vi "AprilTagFieldLayout_New2024.vi"() -> (3 "AprilTagFieldLayout":T1={"AprilTagMap"={}, "FieldLength"=0.0, "FieldWidth"=0.0, "OriginPosition "=enum."kBlueAllianceWallRightSide,", "OriginPose3d"={"Translation3d"={"X"=0.0, "Y"=0.0, "Z"=0.0}, "Rotation3d"={"Q_quaternion"={"R"=1.0, "V"=[0.0, 0.0, 0.0]}}}} {"OriginPose3d"."Translation3d"."Z" format="%14.3f"; "OriginPose3d"."Translation3d"."Y" format="%14.3f"; "OriginPose3d"."Translation3d"."X" format="%14.3f"})   [LabVIEW 2019, in "Trajectory_Library.lvlib"]
doc: "Define the FRC 2024 April Tag field layout.\n\nInputs:\n <none>\n\nOutputs:\n -- AprilTagFieldLayout -- AprilTagFieldLayout -- Data cluster containing field definition."
uses:
  Trajectory_Library.lvlib
  TypeDef/AprilTagFieldLayout.ctl
  TypeDef/AprilTag.ctl
  TypeDef/POSE3D.ctl
  TypeDef/TRANSLATION3D.ctl
  TypeDef/ROTATION3D.ctl
  TypeDef/QUATERNION.ctl
  Enum/AprilTagFieldLayoutOrignPosition_ENUM.ctl
  AprilTag_GetAll.vi
  Quaternion_Normalize.vi
  Quaternion_New_Default.vi
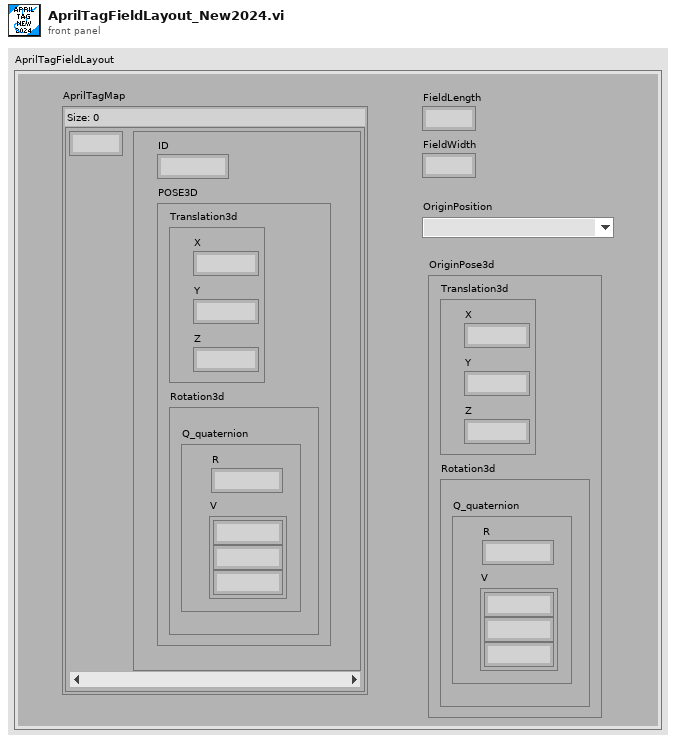
[diagram p1: front panel]
types:
  T1 = typedef "Trajectory_Library.lvlib/AprilTagFieldLayout.ctl" = cluster{"AprilTagMap":map{i32, T2}, "FieldLength":dbl, "FieldWidth":dbl, "OriginPosition ":T7, "OriginPose3d":T3}
  T2 = typedef "Trajectory_Library.lvlib/AprilTag.ctl" = cluster{"ID":i32, "POSE3D":T3}
  T3 = typedef "Trajectory_Library.lvlib/POSE3D.ctl" = cluster{"Translation3d":T4, "Rotation3d":T5}
  T4 = typedef "Trajectory_Library.lvlib/TRANSLATION3D.ctl" = cluster{"X":dbl, "Y":dbl, "Z":dbl}
  T5 = typedef "Trajectory_Library.lvlib/ROTATION3D.ctl" = cluster{"Q_quaternion":T6}
  T6 = typedef "Trajectory_Library.lvlib/QUATERNION.ctl" = cluster{"R":dbl, "V":dbl[]}
  T7 = typedef "Trajectory_Library.lvlib/AprilTagFieldLayoutOrignPosition_ENUM.ctl" = enum16{"kBlueAllianceWallRightSide,", "kRedAllianceWallRightSide,"}
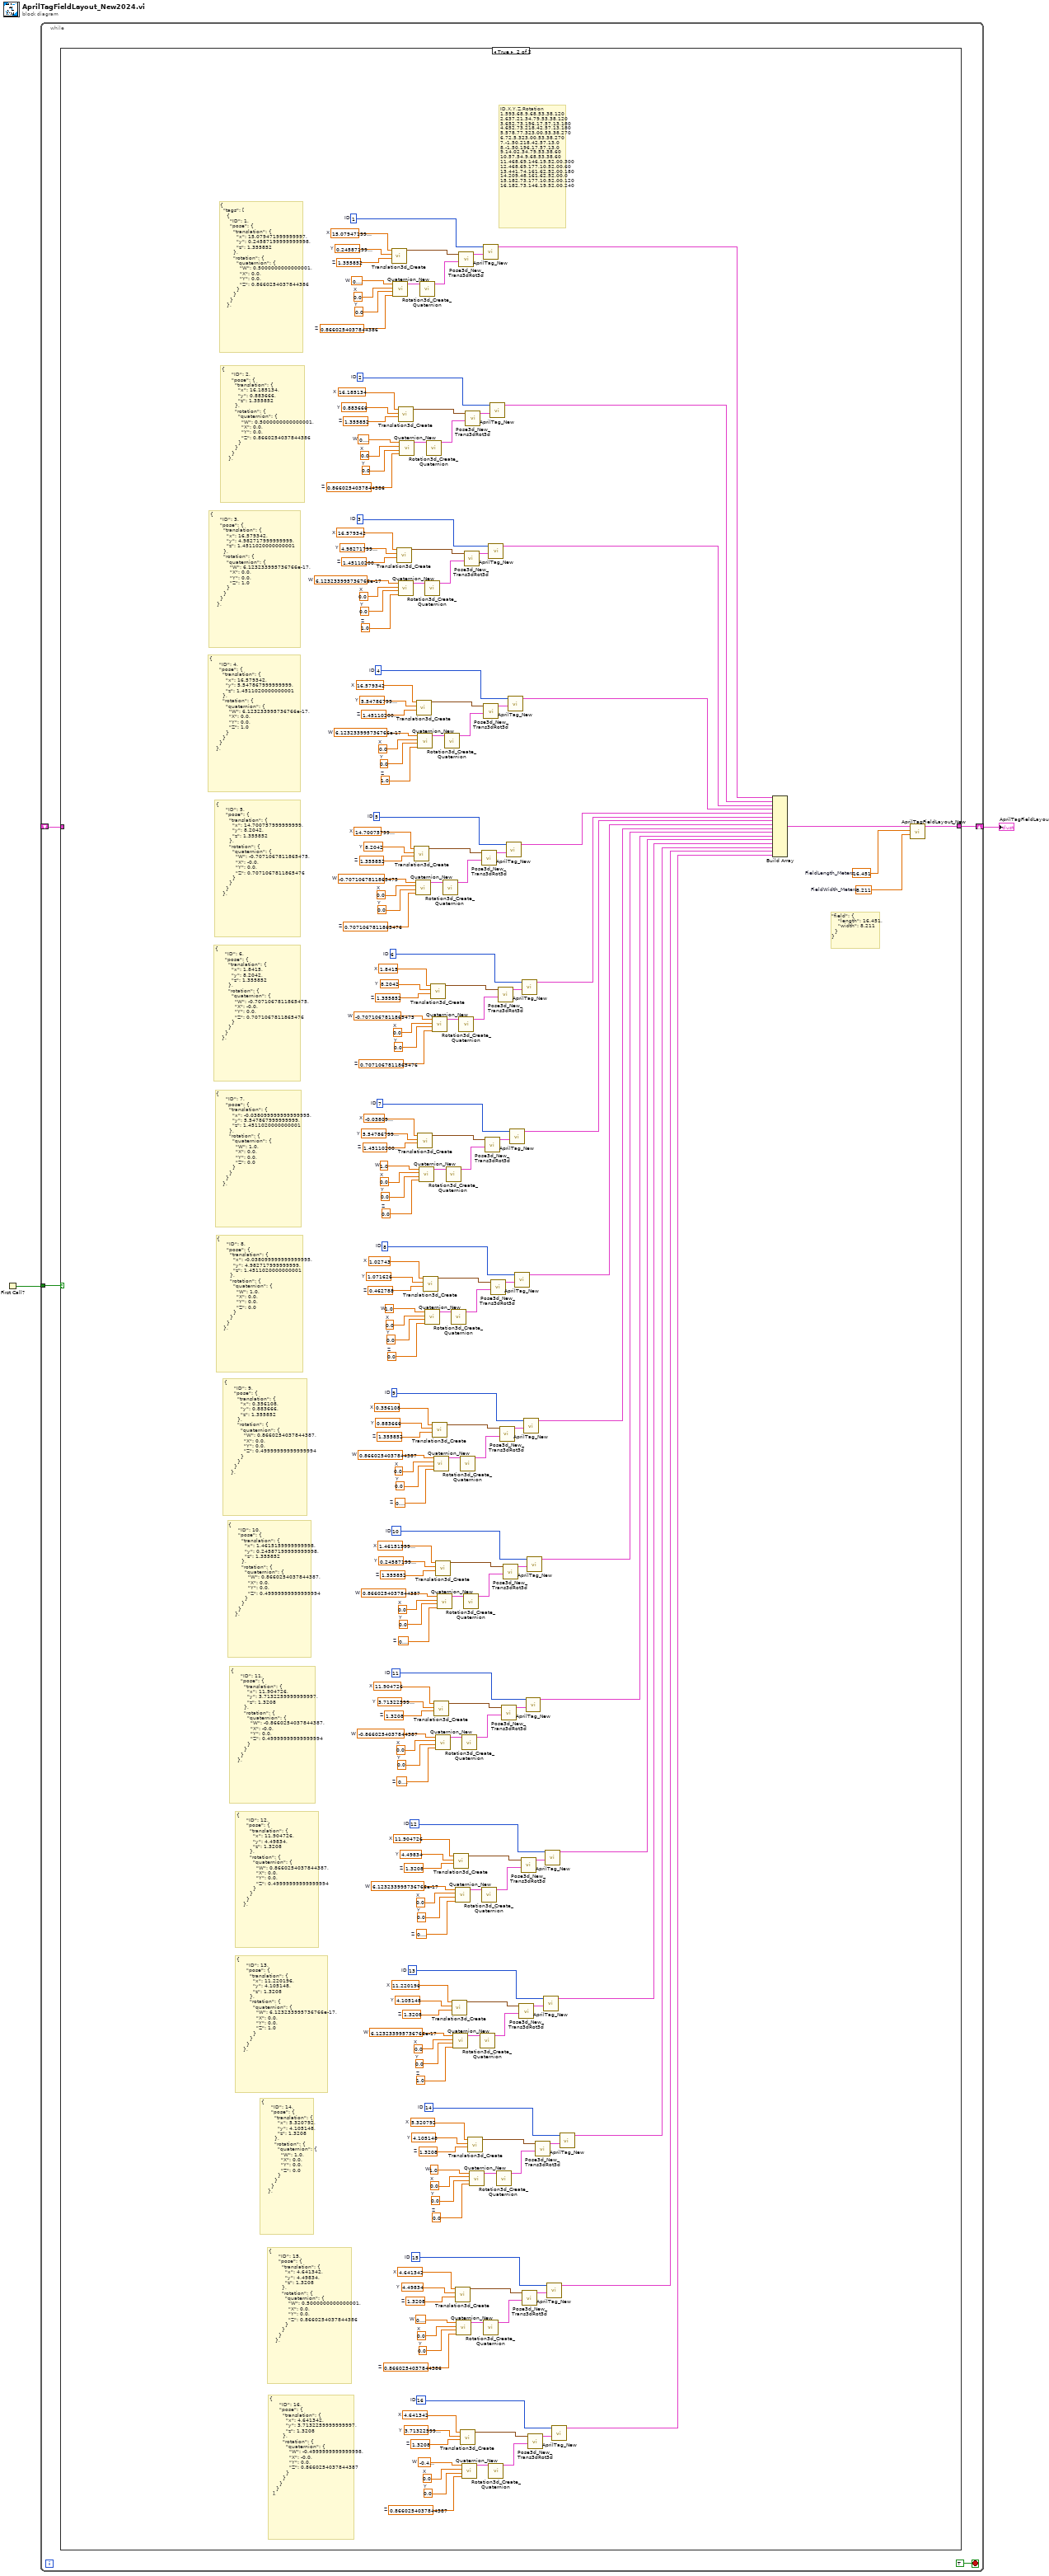
[diagram p0: block diagram]
diagram:
  n1 = First Call?() -> (First Call?: T/F=w1:bool)
  n2 = while {
    shift-right: [w6] -> w2
    shift-left: _ -> [w3]
    tunnel: w1 -> [w4]
    stop <- TRUE stop-if-true
    n3 = case shown="True" w4 {
      tunnel: [w7 w219] -> w6
      tunnel: w3 -> [w7 _]
      frame False {
      }
      frame True {
        w17 = 16  # ID
        w19 = 4.641342  # X
        w20 = 3.7132259999999997  # Y
        w21 = 1.3208  # Z
        w18 = -0.4999999999999998  # W
        w22 = 0.0  # X
        w23 = 0.0  # Y
        w24 = 0.8660254037844387  # Z
        w29 = 15  # ID
        w31 = 4.641342  # X
        w32 = 4.49834  # Y
        w33 = 1.3208  # Z
        w30 = 0.5000000000000001  # W
        w34 = 0.0  # X
        w35 = 0.0  # Y
        w36 = 0.8660254037844386  # Z
        w41 = 14  # ID
        w43 = 5.320792  # X
        w44 = 4.105148  # Y
        w45 = 1.3208  # Z
        w42 = 1.0  # W
        w46 = 0.0  # X
        w47 = 0.0  # Y
        w48 = 0.0  # Z
        w53 = 13  # ID
        w55 = 11.220196  # X
        w56 = 4.105148  # Y
        w57 = 1.3208  # Z
        w54 = 6.123233995736766e-17  # W
        w58 = 0.0  # X
        w59 = 0.0  # Y
        w60 = 1.0  # Z
        w65 = 12  # ID
        w67 = 11.904726  # X
        w68 = 4.49834  # Y
        w69 = 1.3208  # Z
        w66 = 6.123233995736766e-17  # W
        w70 = 0.0  # X
        w71 = 0.0  # Y
        w72 = 0.49999999999999994  # Z
        w77 = 11  # ID
        w79 = 11.904726  # X
        w80 = 3.7132259999999997  # Y
        w81 = 1.3208  # Z
        w78 = -0.8660254037844387  # W
        w82 = 0.0  # X
        w83 = 0.0  # Y
        w84 = 0.49999999999999994  # Z
        w89 = 10  # ID
        w91 = 1.4615159999999998  # X
        w92 = 0.24587199999999998  # Y
        w93 = 1.355852  # Z
        w90 = 0.8660254037844387  # W
        w94 = 0.0  # X
        w95 = 0.0  # Y
        w96 = 0.49999999999999994  # Z
        w101 = 9  # ID
        w103 = 0.356108  # X
        w104 = 0.883666  # Y
        w105 = 1.355852  # Z
        w102 = 0.8660254037844387  # W
        w106 = 0.0  # X
        w107 = 0.0  # Y
        w108 = 0.49999999999999994  # Z
        w122 = 8  # ID
        w124 = 1.02743  # X
        w125 = 1.071626  # Y
        w126 = 0.462788  # Z
        w123 = 1.0  # W
        w127 = 0.0  # X
        w128 = 0.0  # Y
        w129 = 0.0  # Z
        w134 = 7  # ID
        w136 = -0.038099999999999995  # X
        w137 = 5.547867999999999  # Y
        w138 = 1.4511020000000001  # Z
        w135 = 1.0  # W
        w139 = 0.0  # X
        w140 = 0.0  # Y
        w141 = 0.0  # Z
        w146 = 6  # ID
        w148 = 1.8415  # X
        w149 = 8.2042  # Y
        w150 = 1.355852  # Z
        w147 = -0.7071067811865475  # W
        w151 = 0.0  # X
        w152 = 0.0  # Y
        w153 = 0.7071067811865476  # Z
        w158 = 5  # ID
        w160 = 14.700757999999999  # X
        w161 = 8.2042  # Y
        w162 = 1.355852  # Z
        w159 = -0.7071067811865475  # W
        w163 = 0.0  # X
        w164 = 0.0  # Y
        w165 = 0.7071067811865476  # Z
        w170 = 4  # ID
        w172 = 16.579342  # X
        w173 = 5.547867999999999  # Y
        w174 = 1.4511020000000001  # Z
        w171 = 6.123233995736766e-17  # W
        w175 = 0.0  # X
        w176 = 0.0  # Y
        w177 = 1.0  # Z
        w182 = 3  # ID
        w184 = 16.579342  # X
        w185 = 4.982717999999999  # Y
        w186 = 1.4511020000000001  # Z
        w183 = 6.123233995736766e-17  # W
        w187 = 0.0  # X
        w188 = 0.0  # Y
        w189 = 1.0  # Z
        w194 = 2  # ID
        w196 = 16.185134  # X
        w197 = 0.883666  # Y
        w198 = 1.355852  # Z
        w195 = 0.5000000000000001  # W
        w199 = 0.0  # X
        w200 = 0.0  # Y
        w201 = 0.8660254037844386  # Z
        w206 = 1  # ID
        w208 = 15.079471999999997  # X
        w209 = 0.24587199999999998  # Y
        w210 = 1.355852  # Z
        w207 = 0.5000000000000001  # W
        w211 = 0.0  # X
        w212 = 0.0  # Y
        w213 = 0.8660254037844386  # Z
        w217 = 8.211  # FieldWidth_Meters
        w218 = 16.451  # FieldLength_Meters
        # "{\n      \"ID\": 16,\n      \"pose\": {\n        \"translation\": {\n          \"x\": 4.641342,\n          \"y\": 3.7132259999999997,\n          \"z\": 1.3208\n        },\n        \"rotation\": {\n          \"quaternion\": {\n            \"W\": -0.4999999999999998,\n            \"X\": -0.0,\n            \"Y\": 0.0,\n            \"Z\": 0.8660254037844387\n          }\n        }\n      }\n    }\n  ],"
        # "{\n      \"ID\": 15,\n      \"pose\": {\n        \"translation\": {\n          \"x\": 4.641342,\n          \"y\": 4.49834,\n          \"z\": 1.3208\n        },\n        \"rotation\": {\n          \"quaternion\": {\n            \"W\": 0.5000000000000001,\n            \"X\": 0.0,\n            \"Y\": 0.0,\n            \"Z\": 0.8660254037844386\n          }\n        }\n      }\n    },"
        # "{\n      \"ID\": 14,\n      \"pose\": {\n        \"translation\": {\n          \"x\": 5.320792,\n          \"y\": 4.105148,\n          \"z\": 1.3208\n        },\n        \"rotation\": {\n          \"quaternion\": {\n            \"W\": 1.0,\n            \"X\": 0.0,\n            \"Y\": 0.0,\n            \"Z\": 0.0\n          }\n        }\n      }\n    },"
        # "{\n      \"ID\": 13,\n      \"pose\": {\n        \"translation\": {\n          \"x\": 11.220196,\n          \"y\": 4.105148,\n          \"z\": 1.3208\n        },\n        \"rotation\": {\n          \"quaternion\": {\n            \"W\": 6.123233995736766e-17,\n            \"X\": 0.0,\n            \"Y\": 0.0,\n            \"Z\": 1.0\n          }\n        }\n      }\n    },"
        # "{\n      \"ID\": 12,\n      \"pose\": {\n        \"translation\": {\n          \"x\": 11.904726,\n          \"y\": 4.49834,\n          \"z\": 1.3208\n        },\n        \"rotation\": {\n          \"quaternion\": {\n            \"W\": 0.8660254037844387,\n            \"X\": 0.0,\n            \"Y\": 0.0,\n            \"Z\": 0.49999999999999994\n          }\n        }\n      }\n    },"
        # "{\n      \"ID\": 11,\n      \"pose\": {\n        \"translation\": {\n          \"x\": 11.904726,\n          \"y\": 3.7132259999999997,\n          \"z\": 1.3208\n        },\n        \"rotation\": {\n          \"quaternion\": {\n            \"W\": -0.8660254037844387,\n            \"X\": -0.0,\n            \"Y\": 0.0,\n            \"Z\": 0.49999999999999994\n          }\n        }\n      }\n    },"
        # "{\n      \"ID\": 10,\n      \"pose\": {\n        \"translation\": {\n          \"x\": 1.4615159999999998,\n          \"y\": 0.24587199999999998,\n          \"z\": 1.355852\n        },\n        \"rotation\": {\n          \"quaternion\": {\n            \"W\": 0.8660254037844387,\n            \"X\": 0.0,\n            \"Y\": 0.0,\n            \"Z\": 0.49999999999999994\n          }\n        }\n      }\n    },"
        # "{\n      \"ID\": 9,\n      \"pose\": {\n        \"translation\": {\n          \"x\": 0.356108,\n          \"y\": 0.883666,\n          \"z\": 1.355852\n        },\n        \"rotation\": {\n          \"quaternion\": {\n            \"W\": 0.8660254037844387,\n            \"X\": 0.0,\n            \"Y\": 0.0,\n            \"Z\": 0.49999999999999994\n          }\n        }\n      }\n    },"
        # "{\n      \"ID\": 8,\n      \"pose\": {\n        \"translation\": {\n          \"x\": -0.038099999999999995,\n          \"y\": 4.982717999999999,\n          \"z\": 1.4511020000000001\n        },\n        \"rotation\": {\n          \"quaternion\": {\n            \"W\": 1.0,\n            \"X\": 0.0,\n            \"Y\": 0.0,\n            \"Z\": 0.0\n          }\n        }\n      }\n    },"
        # "{\n      \"ID\": 7,\n      \"pose\": {\n        \"translation\": {\n          \"x\": -0.038099999999999995,\n          \"y\": 5.547867999999999,\n          \"z\": 1.4511020000000001\n        },\n        \"rotation\": {\n          \"quaternion\": {\n            \"W\": 1.0,\n            \"X\": 0.0,\n            \"Y\": 0.0,\n            \"Z\": 0.0\n          }\n        }\n      }\n    },"
        # "{\n      \"ID\": 6,\n      \"pose\": {\n        \"translation\": {\n          \"x\": 1.8415,\n          \"y\": 8.2042,\n          \"z\": 1.355852\n        },\n        \"rotation\": {\n          \"quaternion\": {\n            \"W\": -0.7071067811865475,\n            \"X\": -0.0,\n            \"Y\": 0.0,\n            \"Z\": 0.7071067811865476\n          }\n        }\n      }\n    },"
        # "{\n      \"ID\": 5,\n      \"pose\": {\n        \"translation\": {\n          \"x\": 14.700757999999999,\n          \"y\": 8.2042,\n          \"z\": 1.355852\n        },\n        \"rotation\": {\n          \"quaternion\": {\n            \"W\": -0.7071067811865475,\n            \"X\": -0.0,\n            \"Y\": 0.0,\n            \"Z\": 0.7071067811865476\n          }\n        }\n      }\n    },"
        # "{\n      \"ID\": 4,\n      \"pose\": {\n        \"translation\": {\n          \"x\": 16.579342,\n          \"y\": 5.547867999999999,\n          \"z\": 1.4511020000000001\n        },\n        \"rotation\": {\n          \"quaternion\": {\n            \"W\": 6.123233995736766e-17,\n            \"X\": 0.0,\n            \"Y\": 0.0,\n            \"Z\": 1.0\n          }\n        }\n      }\n    },"
        # "{\n      \"ID\": 3,\n      \"pose\": {\n        \"translation\": {\n          \"x\": 16.579342,\n          \"y\": 4.982717999999999,\n          \"z\": 1.4511020000000001\n        },\n        \"rotation\": {\n          \"quaternion\": {\n            \"W\": 6.123233995736766e-17,\n            \"X\": 0.0,\n            \"Y\": 0.0,\n            \"Z\": 1.0\n          }\n        }\n      }\n    },"
        # "{\n      \"ID\": 2,\n      \"pose\": {\n        \"translation\": {\n          \"x\": 16.185134,\n          \"y\": 0.883666,\n          \"z\": 1.355852\n        },\n        \"rotation\": {\n          \"quaternion\": {\n            \"W\": 0.5000000000000001,\n            \"X\": 0.0,\n            \"Y\": 0.0,\n            \"Z\": 0.8660254037844386\n          }\n        }\n      }\n    },"
        # "{\n  \"tags\": [\n    {\n      \"ID\": 1,\n      \"pose\": {\n        \"translation\": {\n          \"x\": 15.079471999999997,\n          \"y\": 0.24587199999999998,\n          \"z\": 1.355852\n        },\n        \"rotation\": {\n          \"quaternion\": {\n            \"W\": 0.5000000000000001,\n            \"X\": 0.0,\n            \"Y\": 0.0,\n            \"Z\": 0.8660254037844386\n          }\n        }\n      }\n    },"
        # "\"field\": {\n    \"length\": 16.451,\n    \"width\": 8.211\n  }\n}"
        # "ID,X,Y,Z,Rotation\n1,593.68,9.68,53.38,120\n2,637.21,34.79,53.38,120\n3,652.73,196.17,57.13,180\n4,652.73,218.42,57.13,180\n5,578.77,323.00,53.38,270\n6,72.5,323.00,53.38,270\n7,-1.50,218.42,57.13,0\n8,-1.50,196.17,57.13,0\n9,14.02,34.79,53.38,60\n10,57.54,9.68,53.38,60\n11,468.69,146.19,52.00,300\n12,468.69,177.10,52.00,60\n13,441.74,161.62,52.00,180\n14,209.48,161.62,52.00,0\n15,182.73,177.10,52.00,120\n16,182.73,146.19,52.00,240"
        n4 = call "Translation3d_Create.vi"("Z"=w210, "Y"=w209, "X"=w208) -> ("TRANSLATION3D"=w216:T4)  [unwired: 8 in]
        n5 = call "Quaternion_New.vi"("Z"=w213, "Y"=w212, "X"=w211, "W"=w207) -> ("out Quaternion"=w214:T6)  [unwired: 7 in]
        n6 = call "Translation3d_Create.vi"("Z"=w186, "Y"=w185, "X"=w184) -> ("TRANSLATION3D"=w192:T4)  [unwired: 8 in]
        n7 = call "Translation3d_Create.vi"("Z"=w198, "Y"=w197, "X"=w196) -> ("TRANSLATION3D"=w204:T4)  [unwired: 8 in]
        n8 = call "Quaternion_New.vi"("Z"=w189, "Y"=w188, "X"=w187, "W"=w183) -> ("out Quaternion"=w190:T6)  [unwired: 7 in]
        n9 = call "Quaternion_New.vi"("Z"=w201, "Y"=w200, "X"=w199, "W"=w195) -> ("out Quaternion"=w202:T6)  [unwired: 7 in]
        n10 = call "Translation3d_Create.vi"("Z"=w162, "Y"=w161, "X"=w160) -> ("TRANSLATION3D"=w168:T4)  [unwired: 8 in]
        n11 = call "Quaternion_New.vi"("Z"=w165, "Y"=w164, "X"=w163, "W"=w159) -> ("out Quaternion"=w166:T6)  [unwired: 7 in]
        n12 = call "Translation3d_Create.vi"("Z"=w174, "Y"=w173, "X"=w172) -> ("TRANSLATION3D"=w180:T4)  [unwired: 8 in]
        n13 = call "Quaternion_New.vi"("Z"=w177, "Y"=w176, "X"=w175, "W"=w171) -> ("out Quaternion"=w178:T6)  [unwired: 7 in]
        n14 = call "Translation3d_Create.vi"("Z"=w138, "Y"=w137, "X"=w136) -> ("TRANSLATION3D"=w144:T4)  [unwired: 8 in]
        n15 = call "Quaternion_New.vi"("Z"=w141, "Y"=w140, "X"=w139, "W"=w135) -> ("out Quaternion"=w142:T6)  [unwired: 7 in]
        n16 = call "Rotation3d_Create_Quaternion.vi"("Quaternion"=w214) -> ("Rotation3d"=w215:T5)  [unwired: 10 in]
        n17 = call "Translation3d_Create.vi"("Z"=w126, "Y"=w125, "X"=w124) -> ("TRANSLATION3D"=w132:T4)  [unwired: 8 in]
        n18 = call "Quaternion_New.vi"("Z"=w129, "Y"=w128, "X"=w127, "W"=w123) -> ("out Quaternion"=w130:T6)  [unwired: 7 in]
        n19 = call "Rotation3d_Create_Quaternion.vi"("Quaternion"=w190) -> ("Rotation3d"=w191:T5)  [unwired: 10 in]
        n20 = call "Rotation3d_Create_Quaternion.vi"("Quaternion"=w202) -> ("Rotation3d"=w203:T5)  [unwired: 10 in]
        n21 = call "Translation3d_Create.vi"("Z"=w150, "Y"=w149, "X"=w148) -> ("TRANSLATION3D"=w156:T4)  [unwired: 8 in]
        n22 = call "Quaternion_New.vi"("Z"=w153, "Y"=w152, "X"=w151, "W"=w147) -> ("out Quaternion"=w154:T6)  [unwired: 7 in]
        n23 = call "Translation3d_Create.vi"("Z"=w105, "Y"=w104, "X"=w103) -> ("TRANSLATION3D"=w111:T4)  [unwired: 8 in]
        n24 = call "Quaternion_New.vi"("Z"=w108, "Y"=w107, "X"=w106, "W"=w102) -> ("out Quaternion"=w109:T6)  [unwired: 7 in]
        n25 = call "Translation3d_Create.vi"("Z"=w81, "Y"=w80, "X"=w79) -> ("TRANSLATION3D"=w87:T4)  [unwired: 8 in]
        n26 = call "Translation3d_Create.vi"("Z"=w93, "Y"=w92, "X"=w91) -> ("TRANSLATION3D"=w99:T4)  [unwired: 8 in]
        n27 = call "Quaternion_New.vi"("Z"=w84, "Y"=w83, "X"=w82, "W"=w78) -> ("out Quaternion"=w85:T6)  [unwired: 7 in]
        n28 = call "Quaternion_New.vi"("Z"=w96, "Y"=w95, "X"=w94, "W"=w90) -> ("out Quaternion"=w97:T6)  [unwired: 7 in]
        n29 = call "Rotation3d_Create_Quaternion.vi"("Quaternion"=w166) -> ("Rotation3d"=w167:T5)  [unwired: 10 in]
        n30 = call "Rotation3d_Create_Quaternion.vi"("Quaternion"=w178) -> ("Rotation3d"=w179:T5)  [unwired: 10 in]
        n31 = call "Rotation3d_Create_Quaternion.vi"("Quaternion"=w142) -> ("Rotation3d"=w143:T5)  [unwired: 10 in]
        n32 = call "Rotation3d_Create_Quaternion.vi"("Quaternion"=w130) -> ("Rotation3d"=w131:T5)  [unwired: 10 in]
        n33 = call "Translation3d_Create.vi"("Z"=w57, "Y"=w56, "X"=w55) -> ("TRANSLATION3D"=w63:T4)  [unwired: 8 in]
        n34 = call "Quaternion_New.vi"("Z"=w60, "Y"=w59, "X"=w58, "W"=w54) -> ("out Quaternion"=w61:T6)  [unwired: 7 in]
        n35 = call "Translation3d_Create.vi"("Z"=w69, "Y"=w68, "X"=w67) -> ("TRANSLATION3D"=w75:T4)  [unwired: 8 in]
        n36 = call "Quaternion_New.vi"("Z"=w72, "Y"=w71, "X"=w70, "W"=w66) -> ("out Quaternion"=w73:T6)  [unwired: 7 in]
        n37 = call "Translation3d_Create.vi"("Z"=w33, "Y"=w32, "X"=w31) -> ("TRANSLATION3D"=w39:T4)  [unwired: 8 in]
        n38 = call "Quaternion_New.vi"("Z"=w36, "Y"=w35, "X"=w34, "W"=w30) -> ("out Quaternion"=w37:T6)  [unwired: 7 in]
        n39 = call "Pose3d_New_Trans3dRot3d.vi"("Rotation3d"=w215, "Translation3d"=w216) -> ("outPose3d"=w205:T3)  [unwired: 9 in]
        n40 = call "Rotation3d_Create_Quaternion.vi"("Quaternion"=w154) -> ("Rotation3d"=w155:T5)  [unwired: 10 in]
        n41 = call "Rotation3d_Create_Quaternion.vi"("Quaternion"=w109) -> ("Rotation3d"=w110:T5)  [unwired: 10 in]
        n42 = call "Translation3d_Create.vi"("Z"=w21, "Y"=w20, "X"=w19) -> ("TRANSLATION3D"=w27:T4)  [unwired: 8 in]
        n43 = call "Quaternion_New.vi"("Z"=w24, "Y"=w23, "X"=w22, "W"=w18) -> ("out Quaternion"=w25:T6)  [unwired: 7 in]
        n44 = call "Rotation3d_Create_Quaternion.vi"("Quaternion"=w85) -> ("Rotation3d"=w86:T5)  [unwired: 10 in]
        n45 = call "Rotation3d_Create_Quaternion.vi"("Quaternion"=w97) -> ("Rotation3d"=w98:T5)  [unwired: 10 in]
        n46 = call "Pose3d_New_Trans3dRot3d.vi"("Rotation3d"=w191, "Translation3d"=w192) -> ("outPose3d"=w181:T3)  [unwired: 9 in]
        n47 = call "Pose3d_New_Trans3dRot3d.vi"("Rotation3d"=w203, "Translation3d"=w204) -> ("outPose3d"=w193:T3)  [unwired: 9 in]
        n48 = call "Translation3d_Create.vi"("Z"=w45, "Y"=w44, "X"=w43) -> ("TRANSLATION3D"=w51:T4)  [unwired: 8 in]
        n49 = call "Quaternion_New.vi"("Z"=w48, "Y"=w47, "X"=w46, "W"=w42) -> ("out Quaternion"=w49:T6)  [unwired: 7 in]
        n50 = call "Rotation3d_Create_Quaternion.vi"("Quaternion"=w61) -> ("Rotation3d"=w62:T5)  [unwired: 10 in]
        n51 = call "Pose3d_New_Trans3dRot3d.vi"("Rotation3d"=w167, "Translation3d"=w168) -> ("outPose3d"=w157:T3)  [unwired: 9 in]
        n52 = call "Rotation3d_Create_Quaternion.vi"("Quaternion"=w73) -> ("Rotation3d"=w74:T5)  [unwired: 10 in]
        n53 = call "AprilTag_New.vi"("POSE3D"=w205, "ID"=w206) -> ("AprilTag"=w119:T2)  [unwired: 9 in]
        n54 = call "Rotation3d_Create_Quaternion.vi"("Quaternion"=w37) -> ("Rotation3d"=w38:T5)  [unwired: 10 in]
        n55 = call "Pose3d_New_Trans3dRot3d.vi"("Rotation3d"=w179, "Translation3d"=w180) -> ("outPose3d"=w169:T3)  [unwired: 9 in]
        n56 = call "Pose3d_New_Trans3dRot3d.vi"("Rotation3d"=w143, "Translation3d"=w144) -> ("outPose3d"=w133:T3)  [unwired: 9 in]
        n57 = call "AprilTag_New.vi"("POSE3D"=w181, "ID"=w182) -> ("AprilTag"=w117:T2)  [unwired: 9 in]
        n58 = call "Rotation3d_Create_Quaternion.vi"("Quaternion"=w25) -> ("Rotation3d"=w26:T5)  [unwired: 10 in]
        n59 = call "AprilTag_New.vi"("POSE3D"=w193, "ID"=w194) -> ("AprilTag"=w118:T2)  [unwired: 9 in]
        n60 = call "Pose3d_New_Trans3dRot3d.vi"("Rotation3d"=w131, "Translation3d"=w132) -> ("outPose3d"=w121:T3)  [unwired: 9 in]
        n61 = call "Rotation3d_Create_Quaternion.vi"("Quaternion"=w49) -> ("Rotation3d"=w50:T5)  [unwired: 10 in]
        n62 = call "Pose3d_New_Trans3dRot3d.vi"("Rotation3d"=w155, "Translation3d"=w156) -> ("outPose3d"=w145:T3)  [unwired: 9 in]
        n63 = call "Pose3d_New_Trans3dRot3d.vi"("Rotation3d"=w110, "Translation3d"=w111) -> ("outPose3d"=w100:T3)  [unwired: 9 in]
        n64 = call "Pose3d_New_Trans3dRot3d.vi"("Rotation3d"=w86, "Translation3d"=w87) -> ("outPose3d"=w76:T3)  [unwired: 9 in]
        n65 = call "Pose3d_New_Trans3dRot3d.vi"("Rotation3d"=w98, "Translation3d"=w99) -> ("outPose3d"=w88:T3)  [unwired: 9 in]
        n66 = call "AprilTag_New.vi"("POSE3D"=w157, "ID"=w158) -> ("AprilTag"=w115:T2)  [unwired: 9 in]
        n67 = call "AprilTag_New.vi"("POSE3D"=w169, "ID"=w170) -> ("AprilTag"=w116:T2)  [unwired: 9 in]
        n68 = call "AprilTag_New.vi"("POSE3D"=w133, "ID"=w134) -> ("AprilTag"=w113:T2)  [unwired: 9 in]
        n69 = call "AprilTag_New.vi"("POSE3D"=w121, "ID"=w122) -> ("AprilTag"=w112:T2)  [unwired: 9 in]
        n70 = call "Pose3d_New_Trans3dRot3d.vi"("Rotation3d"=w62, "Translation3d"=w63) -> ("outPose3d"=w52:T3)  [unwired: 9 in]
        n71 = call "Pose3d_New_Trans3dRot3d.vi"("Rotation3d"=w74, "Translation3d"=w75) -> ("outPose3d"=w64:T3)  [unwired: 9 in]
        n72 = call "AprilTag_New.vi"("POSE3D"=w145, "ID"=w146) -> ("AprilTag"=w114:T2)  [unwired: 9 in]
        n73 = call "Pose3d_New_Trans3dRot3d.vi"("Rotation3d"=w38, "Translation3d"=w39) -> ("outPose3d"=w28:T3)  [unwired: 9 in]
        n74 = call "AprilTag_New.vi"("POSE3D"=w100, "ID"=w101) -> ("AprilTag"=w15:T2)  [unwired: 9 in]
        n75 = call "AprilTag_New.vi"("POSE3D"=w76, "ID"=w77) -> ("AprilTag"=w13:T2)  [unwired: 9 in]
        n76 = call "AprilTag_New.vi"("POSE3D"=w88, "ID"=w89) -> ("AprilTag"=w14:T2)  [unwired: 9 in]
        n77 = call "Pose3d_New_Trans3dRot3d.vi"("Rotation3d"=w26, "Translation3d"=w27) -> ("outPose3d"=w16:T3)  [unwired: 9 in]
        n78 = call "Pose3d_New_Trans3dRot3d.vi"("Rotation3d"=w50, "Translation3d"=w51) -> ("outPose3d"=w40:T3)  [unwired: 9 in]
        n79 = call "AprilTag_New.vi"("POSE3D"=w52, "ID"=w53) -> ("AprilTag"=w11:T2)  [unwired: 9 in]
        n80 = call "AprilTag_New.vi"("POSE3D"=w64, "ID"=w65) -> ("AprilTag"=w12:T2)  [unwired: 9 in]
        n81 = call "AprilTag_New.vi"("POSE3D"=w28, "ID"=w29) -> ("AprilTag"=w9:T2)  [unwired: 9 in]
        n82 = call "AprilTag_New.vi"("POSE3D"=w16, "ID"=w17) -> ("AprilTag"=w8:T2)  [unwired: 9 in]
        n83 = call "AprilTag_New.vi"("POSE3D"=w40, "ID"=w41) -> ("AprilTag"=w10:T2)  [unwired: 9 in]
        n84 = Build Array(w119, w118, w117, w116, w115, w114, w113, w112, w15, w14, w13, w12, w11, w10, w9, w8) -> (w120:T2[])
        n85 = call "AprilTagFieldLayout_New.vi"("FieldWidth_Meters"=w217, "FieldLength_Meters"=w218, "AprilTags"=w120) -> ("AprilTagFieldLayout"=w219:T1)  [unwired: 8 in]
      }
    }
  }
  "AprilTagFieldLayout" <- w2
